vi "Number Format.vi"(9 "기준단위":string, 10 "입력단위":string, 11 "입력값":string) -> (3 "정밀도(단위적용)":i32)   [LabVIEW 2020]
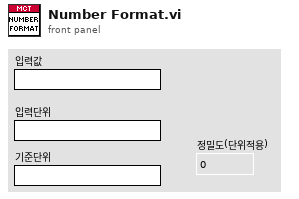
[diagram p1: front panel]
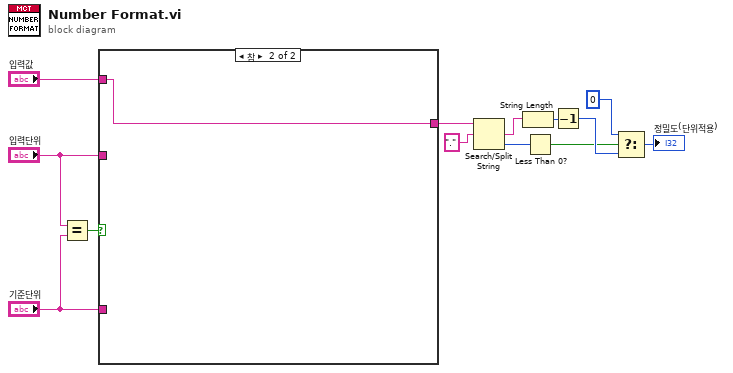
[diagram p0: block diagram]
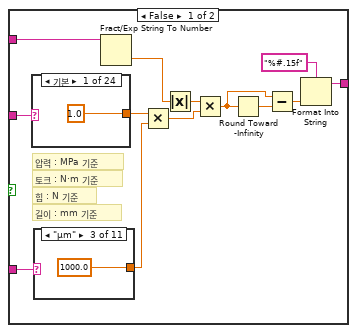
[diagram p2: hidden frame]
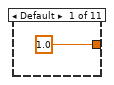
[diagram p3: hidden frame]
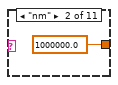
[diagram p4: hidden frame]
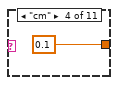
[diagram p5: hidden frame]
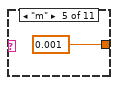
[diagram p6: hidden frame]
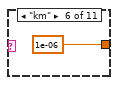
[diagram p7: hidden frame]
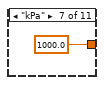
[diagram p8: hidden frame]
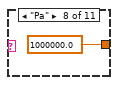
[diagram p9: hidden frame]
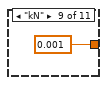
[diagram p10: hidden frame]
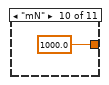
[diagram p11: hidden frame]
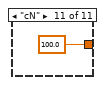
[diagram p12: hidden frame]
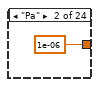
[diagram p13: hidden frame]
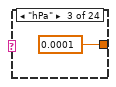
[diagram p14: hidden frame]
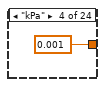
[diagram p15: hidden frame]
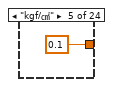
[diagram p16: hidden frame]
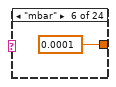
[diagram p17: hidden frame]
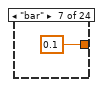
[diagram p18: hidden frame]
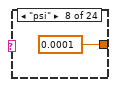
[diagram p19: hidden frame]
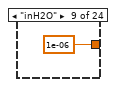
[diagram p20: hidden frame]
diagram:
  n1 = Equal?(x="입력단위", y="기준단위") -> (x = y?=w1:bool)
  n2 = case shown="참" w1 {
    tunnel: "입력값" -> [w25 w62]
    tunnel: [w21 w62] -> w6
    tunnel: "입력단위" -> [w17 _]
    tunnel: "기준단위" -> [w16 _]
    frame False {
      # "길이 : mm 기준"
      # "힘 : N 기준"
      # "토크 : N·m 기준"
      # "압력 : MPa 기준"
      n3 = case shown="기본" w17 {
        tunnel: [1.0 1e-06 0.0001 0.001 0.1 0.0001 0.1 0.0001 1e-06 1e-08 1e-05 0.0001 0.01 1.0 0.0001 0.01 0.001 0.001 1.0 4.0 0.001 0.01 1000.0 10.0] -> w15
        frame Default {
        }
        frame "Pa" {
        }
        frame "hPa" {
        }
        frame "kPa" {
        }
        frame "kgf/㎠" {
        }
        frame "mbar" {
        }
        frame "bar" {
        }
        frame "psi" {
        }
        frame "inH2O" {
        }
        frame "mmH2O" {
        }
        frame "mmHg" {
        }
        frame "inHg" {
        }
        frame "kgf·cm" {
        }
        frame "kgf·m" {
        }
        frame "ozf·in" {
        }
        frame "lbf·ft" {
        }
        frame "cN·m" {
        }
        frame "gf" {
        }
        frame "kgf" {
        }
        frame "lbf" {
        }
        frame "mN" {
        }
        frame "cN" {
        }
        frame "kN" {
        }
        frame "inch" {
        }
      }
      n4 = case shown="\"μm\"" w16 {
        tunnel: [1.0 1000000.0 1000.0 0.1 0.001 1e-06 1000.0 1000000.0 0.001 1000.0 100.0] -> w14
        frame Default {
        }
        frame "nm" {
        }
        frame "μm" {
        }
        frame "cm" {
        }
        frame "m" {
        }
        frame "km" {
        }
        frame "kPa" {
        }
        frame "Pa" {
        }
        frame "kN" {
        }
        frame "mN" {
        }
        frame "cN" {
        }
      }
      n5 = Fract/Exp String To Number(string=w25) -> (number=w19:dbl)  [unwired: 3 in, 1 out]
      n6 = Multiply(x=w15, y=w14) -> (x*y=w26:dbl)
      n7 = Absolute Value(x=w19) -> (abs(x)=w20:dbl)
      n8 = Multiply(x=w20, y=w26) -> (x*y=w24:dbl)
      n9 = Round Toward -Infinity(1:w24) -> (0:w23:dbl)
      n10 = Subtract(x=w24, y=w23) -> (x-y=w22:dbl)
      n11 = Format Into String(format string="%#.15f" ("포맷 문자열"), w22) -> (resulting string=w21:string)  [unwired: 2 in, 1 out]
    }
    frame True {
    }
  }
  n12 = Search/Split String(string=w6, search string/char (-)="." ("검색 문자열/문자 (-)")) -> (match + rest of string=w7:string, offset of match=w9:i32)  [unwired: 1 in, 1 out]
  n13 = String Length(string=w7) -> (length=w8:i32)
  n14 = Less Than 0?(x=w9) -> (x < 0?=w10:bool)
  n15 = Decrement(x=w8) -> (x-1=w11:i32)
  n16 = Select(t=0, s=w10, f=w11) -> (s? t:f=→"정밀도(단위적용)":i32)
